vi "initialize table sizing.vi"(8 "Table in":refnum<vi>, 11 "data type":refnum<vi>) -> ()   [LabVIEW 2013, in "PL Framework Configuration Tool.lvlib" / "EngineTags.lvclass"]
uses:
  EngineTags.lvclass
  <vilib>/NI/Tag Bus/tag/Data Type.ctl
  <vilib>/Utility/miscctls.llb/LVRowAndColumnTypeDef.ctl
  <vilib>/NI/Tag Bus/tag/tag descriptor.lvclass
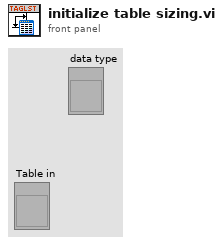
[diagram p1: front panel]
types:
  T1 = typedef "LVRowAndColumnTypeDef.ctl" = cluster{"Row":i32, "Column":i32}
  T2 = typedef "LVBoundsTypeDef.ctl" = cluster{"Width":u32, "Height":u32}
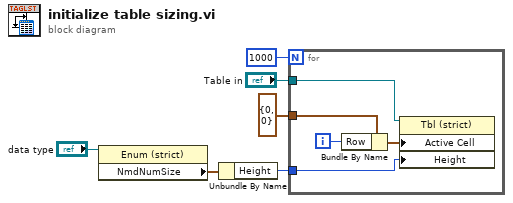
[diagram p0: block diagram]
diagram:
  n1 = property on="Property Node" class="Enum (strict)"(reference="data type") -> ("NmdNumSize"=w6:T2)  [unwired: 1 in, 2 out]
  n2 = Unbundle By Name(w6) -> ("Height"=w4:u32)
  n3 = for {
    N: 1000 -> [_]
    tunnel: T1 {"Row"=0, "Column"=0} ("Active Cell:Active Cell") -> [w11]
    tunnel: "Table in" -> [w8]
    tunnel: w4 -> [w7]
    i -> [w10]
    n4 = Bundle By Name(cluster=w11, "Row"=w10) -> (w9:T1)
    n5 = property on="Property Node" class="Tbl (strict)"(reference=w8, "Active Cell"=w9, "Height"=w7) -> ()  [unwired: 1 in, 2 out]
  }
